vi "StopMusic.vi"(0 "reference in":refnum<class "MediaPlayer.lvclass">, 11 "Error In":errorcluster) -> (4 "reference out":refnum<class "MediaPlayer.lvclass">, 15 "Error Out":errorcluster)   [LabVIEW 2024, in "MediaPlayer.lvclass"]
doc: "Rewind music to start and pause it."
uses:
  MediaPlayer.lvclass
panel:
  # "Connector Pane"
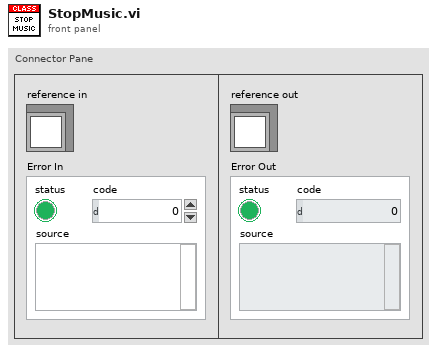
[diagram p1: front panel]
types:
  T1 = typedef "MediaPlayer.lvclass/ObjectAttributes.ctl" = cluster{"MediaPlayerData":T2, "Current Info":T4}
  T2 = typedef "MediaPlayer.lvclass/MediaPlayer Data.ctl" = cluster{"Music List":path[], "Current Music Index":i64, "Song Handler":T3, "Device ID":u32}
  T3 = typedef "Sound Output Task ID.ctl" = u32
  T4 = typedef "MediaPlayer.lvclass/Current Info.ctl" = cluster{"Duration":dbl, "Name":string, "Is playing?":bool, "Current Music Index":i64}
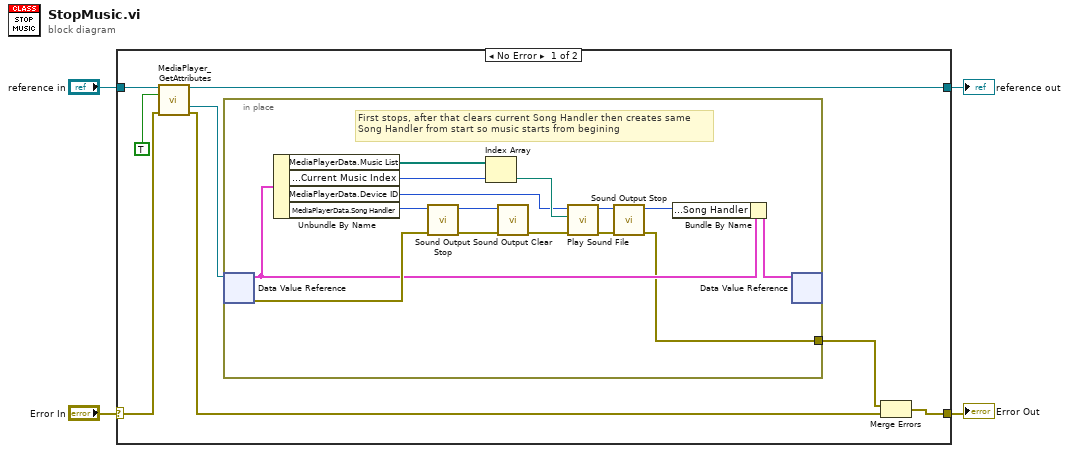
[diagram p0: block diagram]
diagram:
  n1 = case shown="No Error" "Error In" {
    selector: "Error In" -> [w11 w29]
    tunnel: [w6 w29] -> w3
    tunnel: [w10 w28] -> w1
    tunnel: "reference in" -> [w12 w28]
    frame No Error {
      n2 = call "MediaPlayer_GetAttributes.vi"("reference in"=w12, "OnlyGetDvrReference(False)"=TRUE, "Error In"=w11) -> ("reference out"=w10:refnum<class "MediaPlayer.lvclass">, "DataRef"=w7:refnum<data-value>, "Error Out"=w8:errorcluster)  [unwired: 9 in, 1 out]
      n3 = in-place {
        in-place-border: [w15] -> w5
        # "First stops, after that clears current Song Handler then creates same\nSong Handler from start so music starts from begining"
        n4 = in-place-dvr #1(w7) -> (w26:T1, w27:errorcluster)
        n5 = Unbundle By Name(w26) -> ("MediaPlayerData.Music List"=w22:path[], "MediaPlayerData.Current Music Index"=w21:i64, "MediaPlayerData.Device ID"=w17:u32, "MediaPlayerData.Song Handler"=w16:T3)
        n6 = call <vilib>:"Sound Output Stop.vi"("error in (no error)"=w27, "task ID"=w16) -> ("error out"=w20:errorcluster, "task ID out"=w18:T3)  [unwired: 8 in]
        n7 = Index Array(array=w22, index=w21) -> (element=w24:path)
        n8 = call <vilib>:"Sound Output Clear.vi"("error in (no error)"=w20, "task ID"=w18) -> ("error out"=w19:errorcluster)  [unwired: 9 in]
        n9 = call <vilib>:"Play Sound File.vi"("error in (no error)"=w19, "path"=w24, "device ID"=w17) -> ("error out"=w25:errorcluster, "task ID"=w23:T3)  [unwired: 7 in]
        n10 = call <vilib>:"Sound Output Stop.vi"("error in (no error)"=w25, "task ID"=w23) -> ("error out"=w15:errorcluster, "task ID out"=w13:T3)  [unwired: 8 in]
        n11 = Bundle By Name(cluster=w26, "MediaPlayerData.Song Handler"=w13) -> (w14:T1)
        n12 = in-place-dvr #1(w14) -> ()  [unwired: 2 out]
      }
      n13 = Merge Errors(w5, w8) -> (w6:errorcluster)
    }
    frame Error {
    }
  }
  "Error Out" <- w3
  "reference out" <- w1
